vi "WriteCockpitLog.vi"(11 "File In":refnum<file>) -> (3 "File Out":refnum<file>)   [LabVIEW 2010]
uses:
  Subsystems/Global Variables.vi
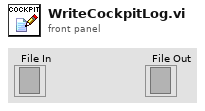
[diagram p1: front panel]
types:
  T1 = cluster{"Accurus button":bool[], "Accurus engaged?":bool, "Vacuum Force":i32, "Accurus Ch. A Vout":dbl, "Accurus Ch. B Vout":dbl, "Irrigation engaged?":bool}
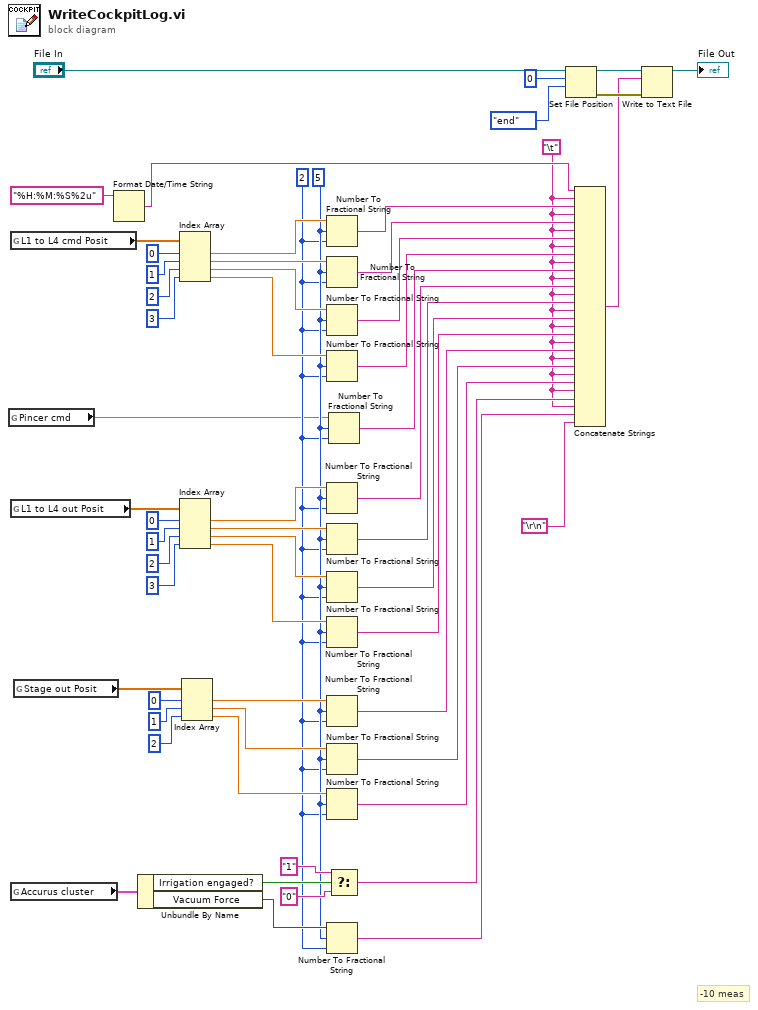
[diagram p0: block diagram]
diagram:
  w8 = 2
  w9 = 5
  w1 = "\t"
  # "-10 meas"
  n1 = global read "Global Variables.vi" "Pincer cmd"() -> (w7:sgl)
  n2 = global read "Global Variables.vi" "L1 to L4 cmd Posit"() -> (w46:dbl[])
  n3 = global read "Global Variables.vi" "L1 to L4 out Posit"() -> (w33:dbl[])
  n4 = global read "Global Variables.vi" "Accurus cluster"() -> (w28:T1)
  n5 = global read "Global Variables.vi" "Stage out Posit"() -> (w21:dbl[])
  n6 = Format Date/Time String(time format string (%c)="%H:%M:%S%2u") -> (date/time string=w10:string)  [unwired: 2 in]
  n7 = Unbundle By Name(w28) -> ("Irrigation engaged?"=w26:bool, "Vacuum Force"=w27:i32)
  n8 = Index Array(array=w46, index #1=0 ("index"), index #2=1 ("index"), index #3=2 ("index"), index #4=3 ("index")) -> (element #1=w45:dbl, element #2=w42:dbl, element #3=w44:dbl, element #4=w43:dbl)
  n9 = Index Array(array=w33, index #1=0 ("index"), index #2=1 ("index"), index #3=2 ("index"), index #4=3 ("index")) -> (element #1=w35:dbl, element #2=w34:dbl, element #3=w40:dbl, element #4=w41:dbl)
  n10 = Index Array(array=w21, index #1=0 ("index"), index #2=1 ("index"), index #3=2 ("index")) -> (element #1=w17:dbl, element #2=w16:dbl, element #3=w15:dbl)
  n11 = Number To Fractional String(number=w45, width (-)=w9, precision (6)=w8) -> (F-format string=w2:string)  [unwired: 1 in]
  n12 = Number To Fractional String(number=w42, width (-)=w9, precision (6)=w8) -> (F-format string=w3:string)  [unwired: 1 in]
  n13 = Number To Fractional String(number=w44, width (-)=w9, precision (6)=w8) -> (F-format string=w4:string)  [unwired: 1 in]
  n14 = Number To Fractional String(number=w43, width (-)=w9, precision (6)=w8) -> (F-format string=w5:string)  [unwired: 1 in]
  n15 = Number To Fractional String(number=w35, width (-)=w9, precision (6)=w8) -> (F-format string=w32:string)  [unwired: 1 in]
  n16 = Number To Fractional String(number=w34, width (-)=w9, precision (6)=w8) -> (F-format string=w31:string)  [unwired: 1 in]
  n17 = Number To Fractional String(number=w40, width (-)=w9, precision (6)=w8) -> (F-format string=w30:string)  [unwired: 1 in]
  n18 = Number To Fractional String(number=w41, width (-)=w9, precision (6)=w8) -> (F-format string=w29:string)  [unwired: 1 in]
  n19 = Number To Fractional String(number=w17, width (-)=w9, precision (6)=w8) -> (F-format string=w14:string)  [unwired: 1 in]
  n20 = Number To Fractional String(number=w16, width (-)=w9, precision (6)=w8) -> (F-format string=w13:string)  [unwired: 1 in]
  n21 = Number To Fractional String(number=w15, width (-)=w9, precision (6)=w8) -> (F-format string=w12:string)  [unwired: 1 in]
  n22 = Number To Fractional String(number=w27, width (-)=w9, precision (6)=w8) -> (F-format string=w23:string)  [unwired: 1 in]
  n23 = Number To Fractional String(number=w7, width (-)=w9, precision (6)=w8) -> (F-format string=w6:string)  [unwired: 1 in]
  n24 = Select(t="1" ("time format string (%c)"), s=w26, f="0" ("time format string (%c)")) -> (s? t:f=w22:string)
  n25 = Set File Position(offset (in bytes) (0)=i64 0, refnum="File In", from (0:start)=enum16{"start", "end", "current"}."end") -> (refnum out=w54:refnum<file>, error out=w53:errorcluster)  [unwired: 1 in]
  n26 = Concatenate Strings(w10, w1, w2, w1, w3, w1, w4, w1, w5, w1, w6, w1, w32, w1, w31, w1, w30, w1, w29, w1, w14, w1, w13, w1, w12, w1, w22, w1, w23, "\r\n") -> (w51:string)
  n27 = Write to Text File(file (use dialog)=w54, text=w51, error in=w53) -> (refnum out=→"File Out":refnum<file>)  [unwired: 1 in, 2 out]
